vi "Day 8.vi"() -> ()   [LabVIEW 2023]
panel:
  out "Grid forest":bool[][](array[boolean])
  out "Answer 2":i32
  out "Answer 1":i16
  in  "test":bool
  in  "test input":string="30373\n25512\n65332\n33549\n35390"
  in  "input":string="003112220410413101104044022234320204233341435252223642044225451531421012104343030211442433410302111\n301233004003313130222434121135033231250505241131342032404032560542233000343455552123100410402211201\n111301041221333142533352050250154136146324550411565615444115604102531135302000320033233340431313123\n011312210420442043155233305201305643445224334303310253225205601265233454400214114322131420224022313\n130102441231200141254202121022423405224443210463250415204410624313613034320040015223211432442333110\n133121132322223054104323242043651144066341346000104210124535555236324451132555525220523220023202433\n..."
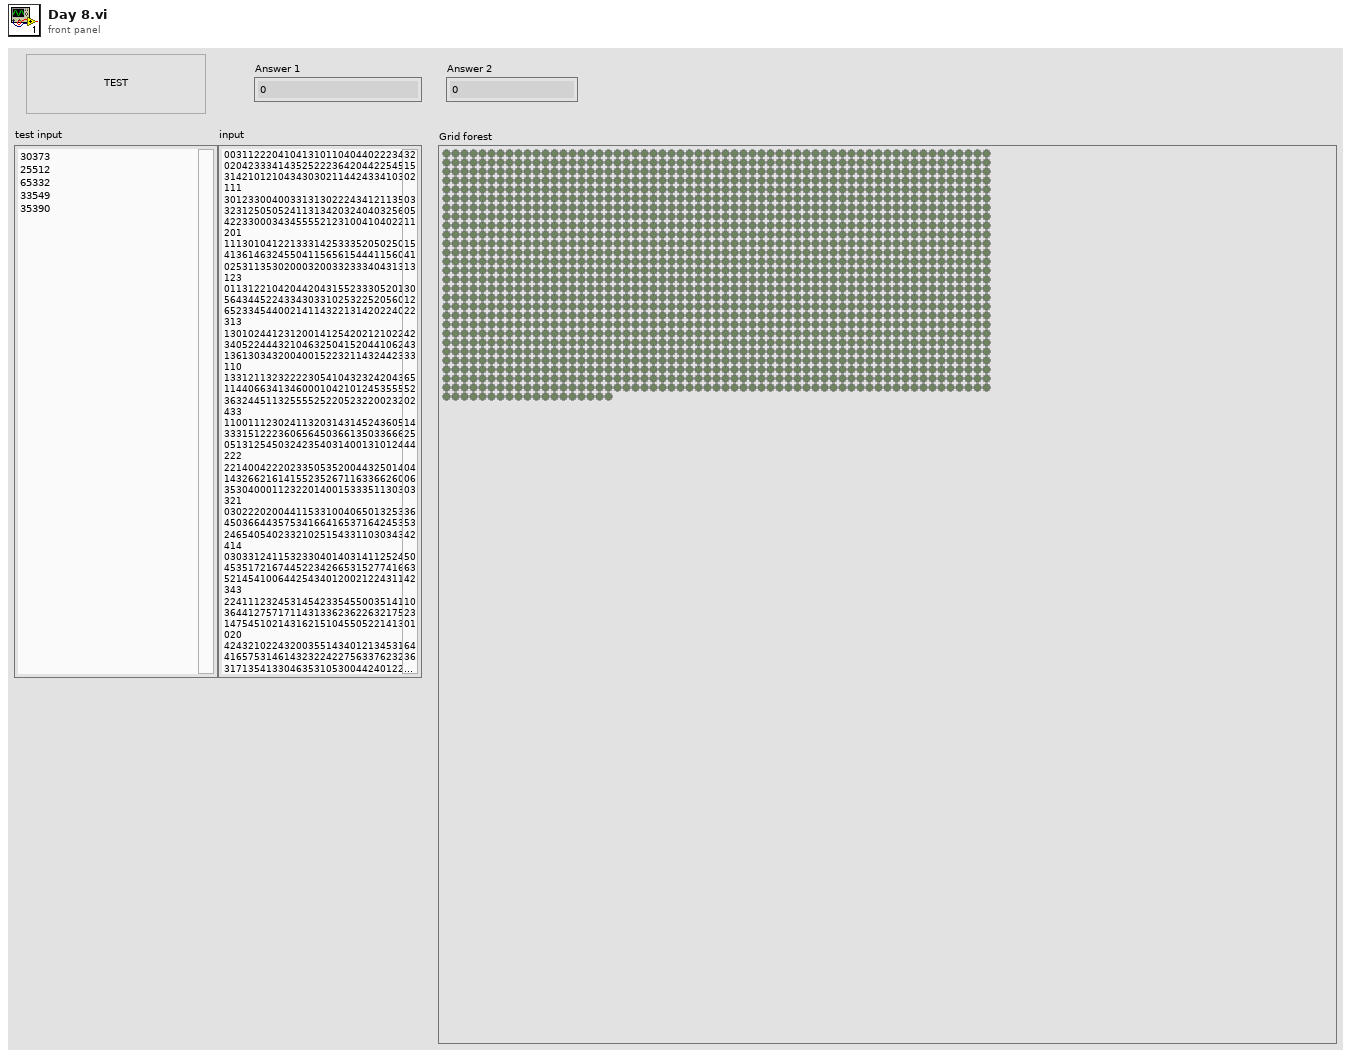
[diagram p1: front panel]
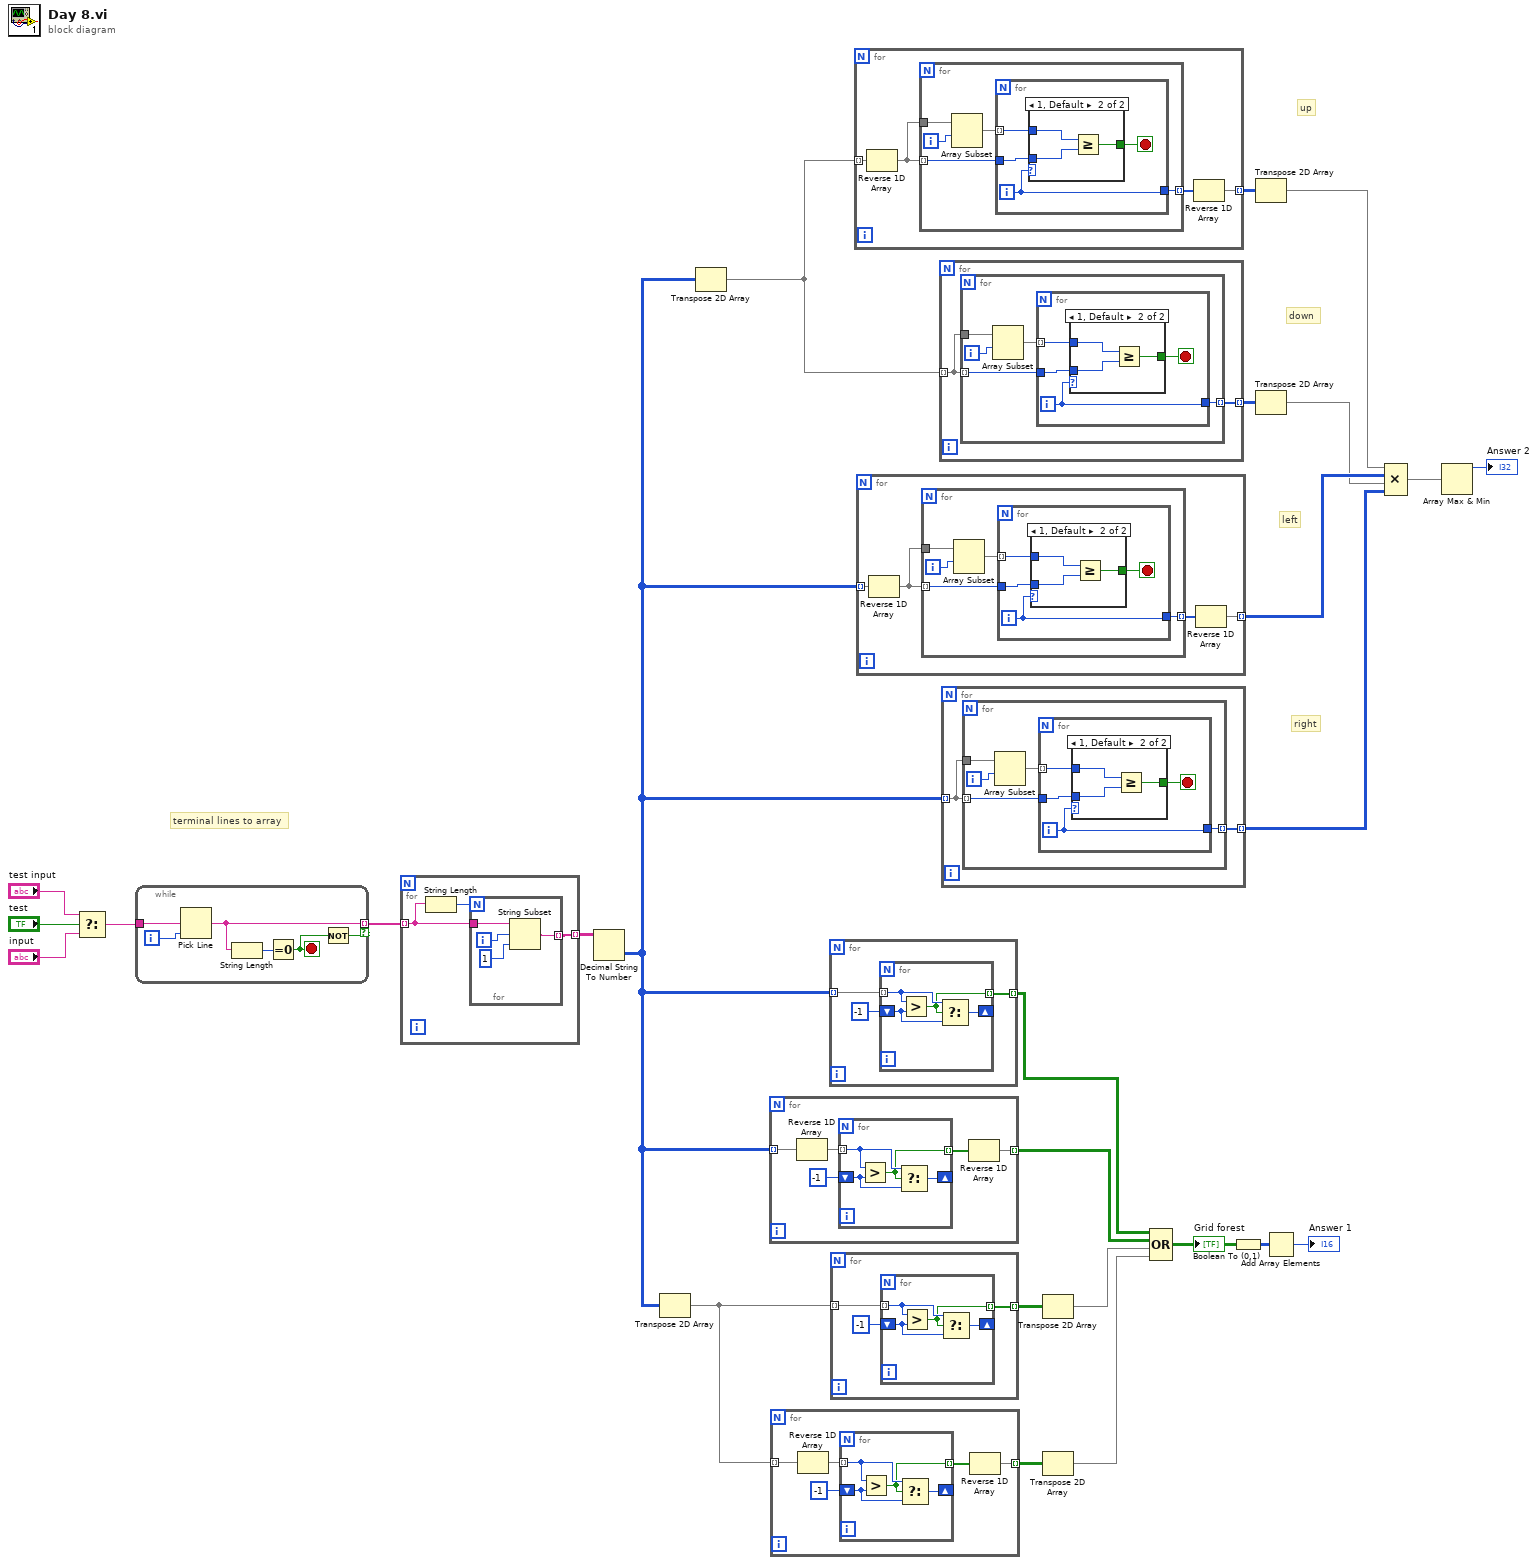
[diagram p0: block diagram]
diagram:
  # "right"
  # "left"
  # "down"
  # "up"
  # "terminal lines to array"
  n1 = Select(t="test input", s="test", f="input") -> (s? t:f=w25:string)
  n2 = while {
    tunnel: w25 -> [w30]
    tunnel: [w29] -> w22 mode=indexing if=w27
    i -> [w31]
    stop <- w28 stop-if-true
    n3 = Pick Line(multi-line string=w30, line index=w31) -> (output string=w29:string)  [unwired: 1 in]
    n4 = String Length(string=w29) -> (length=w32:i32)
    n5 = Equal To 0?(x=w32) -> (x = 0?=w28:bool)
    n6 = Not(x=w28) -> (.not. x?=w27:bool)
  }
  n7 = for {
    tunnel: w22 -> [w34] mode=indexing
    tunnel: [w33] -> w21 mode=indexing
    n8 = String Length(string=w34) -> (length=w35:i32)
    n9 = for {
      N: w35 -> [_]
      tunnel: w34 -> [w37]
      tunnel: [w36] -> w33 mode=indexing
      i -> [w39]
      n10 = String Subset(string=w37, offset (0)=w39, length (rest)=1 ("length (rest)")) -> (substring=w36:string)
    }
  }
  n11 = Decimal String To Number(string=w21) -> (number=w7:i32[][])  [unwired: 2 in, 1 out]
  n12 = Transpose 2D Array(2D array=w7) -> (transposed array=w14:i32[][])
  n13 = Transpose 2D Array(2D array=w7) -> (transposed array=w6:i32[][])
  n14 = for {
    tunnel: w7 -> [w44] mode=indexing
    tunnel: [w40] -> w20 mode=indexing
    n15 = Reverse 1D Array(array=w44) -> (reversed array=w41:i32[])
    n16 = for {
      tunnel: w41 -> [w47] mode=indexing
      shift-right: [w48] -> _
      shift-left: -1 ("output string") -> [w46]
      tunnel: [w45] -> w42 mode=indexing
      n17 = Greater?(x=w47, y=w46) -> (0:w45:bool)
      n18 = Select(t=w47, s=w45, f=w46) -> (s? t:f=w48:i32)
    }
    n19 = Reverse 1D Array(array=w42) -> (reversed array=w40:bool[])
  }
  n20 = for {
    tunnel: w14 -> [w53] mode=indexing
    tunnel: [w49] -> w15 mode=indexing
    n21 = Reverse 1D Array(array=w53) -> (reversed array=w50:i32[])
    n22 = for {
      tunnel: w50 -> [w56] mode=indexing
      shift-right: [w57] -> _
      shift-left: -1 ("output string") -> [w55]
      tunnel: [w54] -> w51 mode=indexing
      n23 = Greater?(x=w56, y=w55) -> (0:w54:bool)
      n24 = Select(t=w56, s=w54, f=w55) -> (s? t:f=w57:i32)
    }
    n25 = Reverse 1D Array(array=w51) -> (reversed array=w49:bool[])
  }
  n26 = for {
    tunnel: w7 -> [w60] mode=indexing
    tunnel: [w58] -> w17 mode=indexing
    n27 = for {
      tunnel: w60 -> [w63] mode=indexing
      shift-right: [w64] -> _
      shift-left: -1 ("output string") -> [w62]
      tunnel: [w61] -> w58 mode=indexing
      n28 = Greater?(x=w63, y=w62) -> (0:w61:bool)
      n29 = Select(t=w63, s=w61, f=w62) -> (s? t:f=w64:i32)
    }
  }
  n30 = for {
    tunnel: w14 -> [w67] mode=indexing
    tunnel: [w65] -> w16 mode=indexing
    n31 = for {
      tunnel: w67 -> [w70] mode=indexing
      shift-right: [w71] -> _
      shift-left: -1 ("output string") -> [w69]
      tunnel: [w68] -> w65 mode=indexing
      n32 = Greater?(x=w70, y=w69) -> (0:w68:bool)
      n33 = Select(t=w70, s=w68, f=w69) -> (s? t:f=w71:i32)
    }
  }
  n34 = for {
    tunnel: w6 -> [w75] mode=indexing
    tunnel: [w72] -> w8 mode=indexing
    n35 = Reverse 1D Array(array=w75) -> (reversed array=w73:i32[])
    n36 = for {
      tunnel: w73 -> [w80] mode=indexing
      tunnel: w73 -> [w79]
      tunnel: [w77] -> w74 mode=indexing
      i -> [w76]
      n37 = Array Subset(array=w79, index=w76) -> (w78:i32[])  [unwired: 1 in]
      n38 = for {
        tunnel: w80 -> [w84]
        tunnel: w78 -> [w83] mode=indexing
        tunnel: [w81] -> w77
        i -> [w81]
        stop <- w82 stop-if-true
        n39 = case shown="1, Default" w81 {
          tunnel: w84 -> [_ w87]
          tunnel: w83 -> [_ w86]
          tunnel: [_ w85] -> w82
          frame 0 {
          }
          frame 1, Default {
            n40 = Greater Or Equal?(x=w86, y=w87) -> (x >= y?=w85:bool)
          }
        }
      }
    }
    n41 = Reverse 1D Array(array=w74) -> (reversed array=w72:i32[])
  }
  n42 = for {
    tunnel: w7 -> [w91] mode=indexing
    tunnel: [w88] -> w4 mode=indexing
    n43 = Reverse 1D Array(array=w91) -> (reversed array=w89:i32[])
    n44 = for {
      tunnel: w89 -> [w96] mode=indexing
      tunnel: w89 -> [w95]
      tunnel: [w93] -> w90 mode=indexing
      i -> [w92]
      n45 = Array Subset(array=w95, index=w92) -> (w94:i32[])  [unwired: 1 in]
      n46 = for {
        tunnel: w96 -> [w100]
        tunnel: w94 -> [w99] mode=indexing
        tunnel: [w97] -> w93
        i -> [w97]
        stop <- w98 stop-if-true
        n47 = case shown="1, Default" w97 {
          tunnel: w100 -> [_ w103]
          tunnel: w99 -> [_ w102]
          tunnel: [_ w101] -> w98
          frame 0 {
          }
          frame 1, Default {
            n48 = Greater Or Equal?(x=w102, y=w103) -> (x >= y?=w101:bool)
          }
        }
      }
    }
    n49 = Reverse 1D Array(array=w90) -> (reversed array=w88:i32[])
  }
  n50 = for {
    tunnel: w6 -> [w105] mode=indexing
    tunnel: [w104] -> w9 mode=indexing
    n51 = for {
      tunnel: w105 -> [w110] mode=indexing
      tunnel: w105 -> [w109]
      tunnel: [w107] -> w104 mode=indexing
      i -> [w106]
      n52 = Array Subset(array=w109, index=w106) -> (w108:i32[])  [unwired: 1 in]
      n53 = for {
        tunnel: w110 -> [w114]
        tunnel: w108 -> [w113] mode=indexing
        tunnel: [w111] -> w107
        i -> [w111]
        stop <- w112 stop-if-true
        n54 = case shown="1, Default" w111 {
          tunnel: w114 -> [_ w117]
          tunnel: w113 -> [_ w116]
          tunnel: [_ w115] -> w112
          frame 0 {
          }
          frame 1, Default {
            n55 = Greater Or Equal?(x=w116, y=w117) -> (x >= y?=w115:bool)
          }
        }
      }
    }
  }
  n56 = for {
    tunnel: w7 -> [w119] mode=indexing
    tunnel: [w118] -> w10 mode=indexing
    n57 = for {
      tunnel: w119 -> [w124] mode=indexing
      tunnel: w119 -> [w123]
      tunnel: [w121] -> w118 mode=indexing
      i -> [w120]
      n58 = Array Subset(array=w123, index=w120) -> (w122:i32[])  [unwired: 1 in]
      n59 = for {
        tunnel: w124 -> [w128]
        tunnel: w122 -> [w127] mode=indexing
        tunnel: [w125] -> w121
        i -> [w125]
        stop <- w126 stop-if-true
        n60 = case shown="1, Default" w125 {
          tunnel: w128 -> [_ w131]
          tunnel: w127 -> [_ w130]
          tunnel: [_ w129] -> w126
          frame 0 {
          }
          frame 1, Default {
            n61 = Greater Or Equal?(x=w130, y=w131) -> (x >= y?=w129:bool)
          }
        }
      }
    }
  }
  n62 = Transpose 2D Array(2D array=w16) -> (transposed array=w13:bool[][])
  n63 = Transpose 2D Array(2D array=w15) -> (transposed array=w12:bool[][])
  n64 = Compound Arithmetic op=OR(w17, w20, w13, w12) -> (w19:bool[][])
  "Grid forest" <- w19
  n65 = Boolean To (0,1)(Boolean=w19) -> (0, 1=w18:i16[][])
  n66 = Transpose 2D Array(2D array=w8) -> (transposed array=w5:i32[][])
  n67 = Transpose 2D Array(2D array=w9) -> (transposed array=w3:i32[][])
  n68 = Add Array Elements(numeric array=w18) -> (sum=→"Answer 1":i16)
  n69 = Compound Arithmetic op=MULTIPLY(w5, w4, w3, w10) -> (w1:i32[][])
  n70 = Array Max & Min(array=w1) -> (max value=→"Answer 2":i32)  [unwired: 3 out]
